vi "GetDisplayData.vi"(8 "error in":errorcluster caption="错误输入（无错误）", 11 "Display Config":T1={"Display Mode"=enum."时域", "ChTag[]"=[], "window"=1, "Range"={"Minimum"=0.0, "Maximum"=0.0, "Increment"=0.0, "Minor Increment"=0.0, "Start"=0.0}} {"window" items=["Rectangle"=0, "Hanning"=1, "Hamming"=2, "Blackman-Harris"=3, "Exact Blackman"=4, "Blackman"=5, "Flat Top"=6, "4 Term B-Harris "=7, "7 Term B-Harris"=8, "Low Sidelobe"=9, "Blackman Nuttall"=11, "Triangle"=30, "Bartlett-Hanning"=31, "Bohman"=32, "Parzen"=33, "Welch"=34, "Kaiser"=60, "Dolph-Chebyshev"=61, "Gaussian"=62]}) -> (0 "error out":errorcluster caption="错误输出", 1 "Data":cluster{"f0":dbl, "df":dbl, "magnitude":dbl[]}[](array[cluster]), 2 "Valid?":bool)   [LabVIEW 2016]
uses:
  Display Config.ctl
  Display Mode.ctl
  <vilib>/Analysis/4window.llb/windowTd.ctl
  <vilib>/Utility/miscctls.llb/LVRangeTypeDef.ctl
  <vilib>/measure/maspectr.llb/FFT Spectrum (Mag-Phase) for N Chan.vi
  <vilib>/measure/maspectr.llb/FFT Power Spectrum and PSD for N Chan.vi
  <vilib>/measure/NI_MAPro.lvlib
  PCM PanelSplit.lvclass
  <vilib>/Analysis/NI_AALPro.lvlib
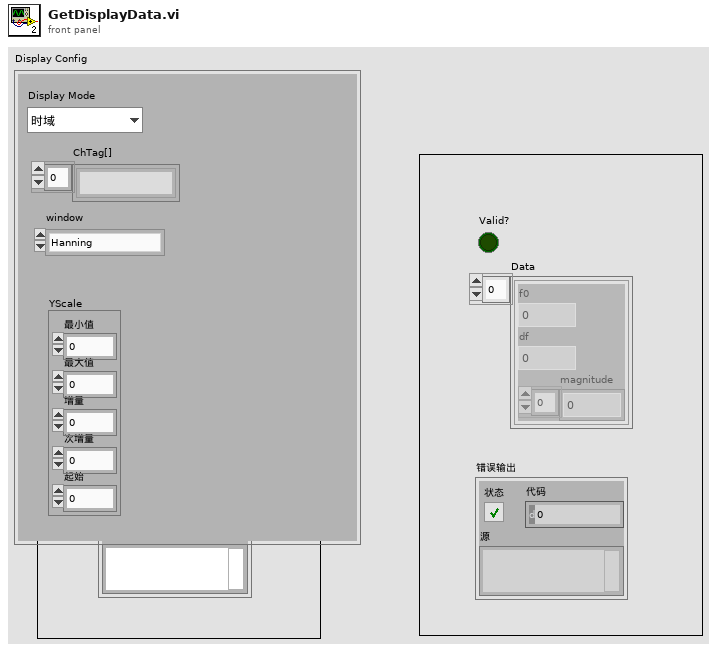
[diagram p1: front panel]
types:
  T1 = typedef "PCM PanelSplit.lvclass/Display Config.ctl" = cluster{"Display Mode":T2, "ChTag[]":string[], "window":T3, "Range":T4}
  T2 = typedef "PCM PanelSplit.lvclass/Display Mode.ctl" = enum16{"时域", "频谱", "功率谱"}
  T3 = typedef "NI_AALPro.lvlib/windowTd.ctl" = u32
  T4 = typedef "LVRangeTypeDef.ctl" = cluster{"Minimum":dbl, "Maximum":dbl, "Increment":dbl, "Minor Increment":dbl, "Start":dbl}
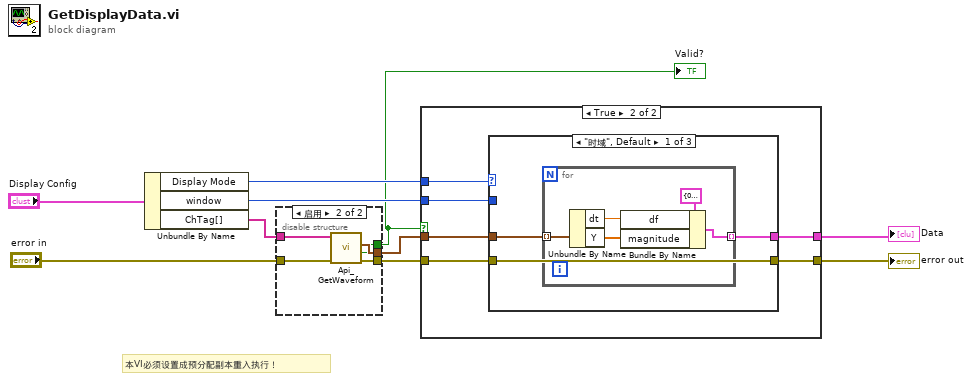
[diagram p0: block diagram]
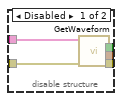
[diagram p2: hidden frame]
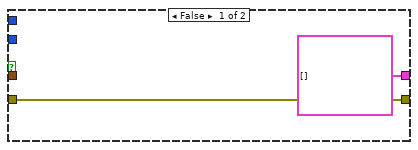
[diagram p3: hidden frame]
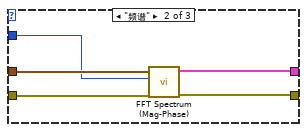
[diagram p4: hidden frame]
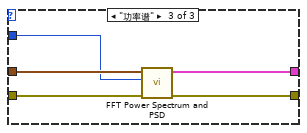
[diagram p5: hidden frame]
diagram:
  # "本VI必须设置成预分配副本重入执行！"
  n1 = Unbundle By Name("Display Config") -> ("Display Mode"=w5:T2, "window"=w6:T3, "ChTag[]"=w9:string[])
  n2 = disable-structure shown="启用" {
    disable-tunnel: w9 -> [w15 w16]
    disable-tunnel: "error in" -> [w14 w17]
    disable-tunnel: [w13 w19] -> w1
    disable-tunnel: [w12 w20] -> w7
    disable-tunnel: [w11 w18] -> w4
    frame Disabled {
      n3 = call "GetWaveform.vi"("error in (no error)"=w14, "ChannelTag[]"=w15) -> ("error out"=w11:errorcluster, "Waveform"=w12:waveform(dbl)[], "Valid?"=w13:bool)  [unwired: 7 in]
    }
    frame Enabled {
      n4 = call "Api_GetWaveform.vi"("error in (no error)"=w17, "Tags[]"=w16) -> ("error out"=w18:errorcluster, "Display?"=w19:bool, "Wave[]"=w20:waveform(dbl)[])  [unwired: 7 in]
    }
  }
  "Valid?" <- w1
  n5 = case shown="True" w1 {
    tunnel: w7 -> [_ w26]
    tunnel: w6 -> [_ w27]
    tunnel: w5 -> [_ w28]
    tunnel: [cluster{"f0":dbl, "df":dbl, "magnitude":dbl[]}[] [] ("Power Spectrum / PSD") w25] -> w2
    tunnel: w4 -> [w22 w24]
    tunnel: [w22 w23] -> w3
    frame False {
    }
    frame True {
      n6 = case shown="\"时域\", Default" w28 {
        tunnel: w27 -> [_ w37 w45]
        tunnel: w26 -> [w30 w39 w46]
        tunnel: [w29 w38 w44] -> w25
        tunnel: w24 -> [w31 w41 w43]
        tunnel: [w31 w40 w42] -> w23
        frame "时域", Default {
          n7 = for {
            tunnel: w30 -> [w36] mode=indexing
            tunnel: [w32] -> w29 mode=indexing
            n8 = Unbundle By Name(w36) -> ("dt"=w34:dbl, "Y"=w33:dbl[])
            n9 = Bundle By Name(cluster=cluster{"f0":dbl, "df":dbl, "magnitude":dbl[]} {"f0"=0.0, "df"=0.0, "magnitude"=[]} ("power spectrum"), "df"=w34, "magnitude"=w33) -> (w32:cluster{"f0":dbl, "df":dbl, "magnitude":dbl[]})
          }
        }
        frame "频谱" {
          n10 = call-poly <vilib>:"FFT Spectrum (Mag-Phase).vi"("error in (no error)"=w41, "window"=w37, "time signals"=w39) -> ("error out"=w40:errorcluster, "magnitudes"=w38:cluster{"f0":dbl, "df":dbl, "magnitude":dbl[]}[])  [unwired: 4 in, 3 out]
        }
        frame "功率谱" {
          n11 = call-poly <vilib>:"FFT Power Spectrum and PSD.vi"("error in (no error)"=w43, "window"=w45, "time signals"=w46) -> ("error out"=w42:errorcluster, "Power Spectrum / PSD"=w44:cluster{"f0":dbl, "df":dbl, "magnitude":dbl[]}[])  [unwired: 5 in, 2 out]
        }
      }
    }
  }
  "error out" <- w3
  "Data" <- w2
